vi "Push New Tone.vi"(8 "error in (no error)":errorcluster, 10 "signal":waveform(dbl), 11 "Receiver in":refnum<class "Receiver.lvclass">) -> (0 "error out":errorcluster, 3 "Receiver out":refnum<class "Receiver.lvclass">)   [LabVIEW 2013, in "Receiver.lvclass"]
uses:
  Receiver.lvclass
  Receiver.lvclass/Receiver.ctl
panel:
  out "sync?":bool
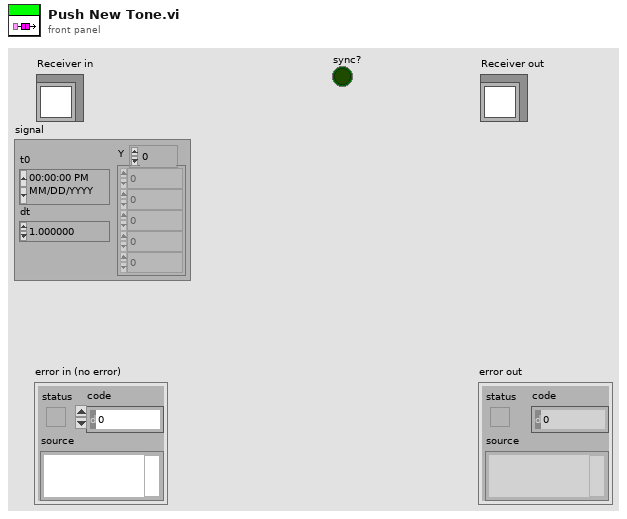
[diagram p1: front panel]
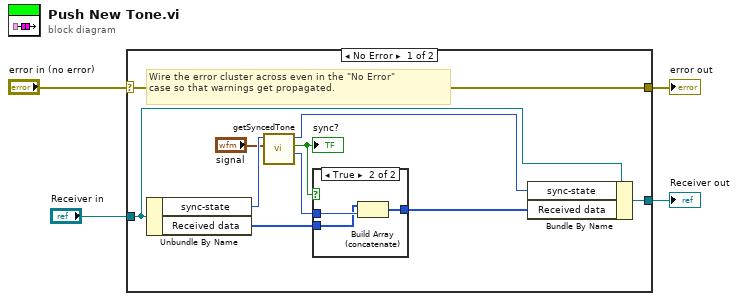
[diagram p0: block diagram]
diagram:
  n1 = case shown="No Error" "error in (no error)" {
    selector: "error in (no error)" -> [w14 w20]
    tunnel: [w14 w20] -> w3
    tunnel: [w12 w19] -> w1
    tunnel: "Receiver in" -> [w13 w19]
    frame No Error {
      # "Wire the error cluster across even in the \"No Error\"\ncase so that warnings get propagated."
      n2 = Unbundle By Name(w13) -> ("sync-state"=w11:enum16{"not-sync", "synced"}, "Received data"=w7:i32[])
      n3 = call "getSyncedTone.vi"("signal"="signal", "sync-state"=w11) -> ("tone"=w8:i32, "sync?"=w9:bool, "sync-state"=w10:enum16{"not-sync", "synced"})  [unwired: 6 in, 1 out]
      "sync?" <- w9
      n4 = case shown="True" w9 {
        tunnel: w8 -> [_ w18]
        tunnel: w7 -> [w15 w17]
        tunnel: [w15 w16] -> w5
        frame False {
        }
        frame True {
          n5 = Build Array (concatenate)(w17, w18) -> (w16:i32[])
        }
      }
      n6 = Bundle By Name(cluster=w13, "sync-state"=w10, "Received data"=w5) -> (w12:refnum<class "Receiver.lvclass">)
    }
    frame Error {
    }
  }
  "error out" <- w3
  "Receiver out" <- w1
